vi "Host Main.vi"() -> ()   [LabVIEW 2013]
doc: "This application launches and executes the Tag Bus Data framework configuration for the specified target alias. This is a simple example of the framework API functions, but may also be a suitable starting point for a Host UI or Thick Client that is running a local version of the framework."
uses:
  <vilib>/NI/Module Execution Interface/Engine Runtime/Execution States.ctl
  <vilib>/NI/Module Execution Interface/Engine Runtime/Fault.ctl
  <vilib>/NI/Tag Bus Module Framework/runtime/error classification.ctl
  <vilib>/NI/Module Execution Interface/Engine Runtime/Engine Runtime Interface.lvclass
  <vilib>/NI/Tag Bus Data Framework/Framework Configuration Classes/target runtime/PL_Target Runtime.lvclass
  <vilib>/NI/Tag Bus Module Framework/runtime/TBM module execution interface.lvclass
panel:
  out "engine status":T4(array[cluster])
  in  "file name":string="SimulatedSystem.pcfg"
  in  "stop":bool
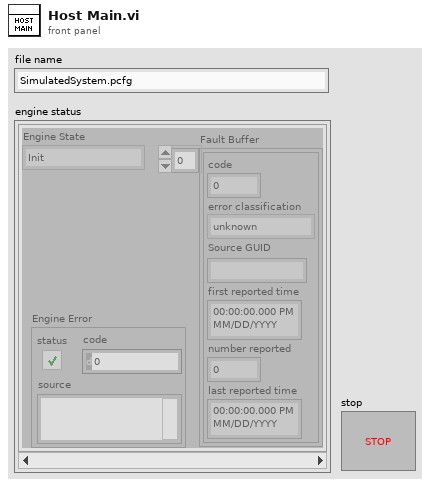
[diagram p1: front panel]
types:
  T1 = typedef "Engine Runtime Interface.lvclass/Execution States.ctl" = enum16{"Init", "Pre-Operational", "Safe-Operational", "Operational", "Stopped"}
  T2 = typedef "Engine Runtime Interface.lvclass/Fault.ctl" = cluster{"code":i32, "error classification":T3, "Source GUID":string, "first reported time":timestamp, "number reported":u32, "last reported time":timestamp}
  T3 = typedef "TBM module execution interface.lvclass/error classification.ctl" = enum16{"unknown", "none", "trivial", "recoverable", "critical"}
  T4 = cluster{"Engine State":T1, "Fault Buffer":T2[], "Engine Error":errorcluster}[]
  T5 = cluster{"Engine State":T1, "faults":T2[], "Engine Error":errorcluster}
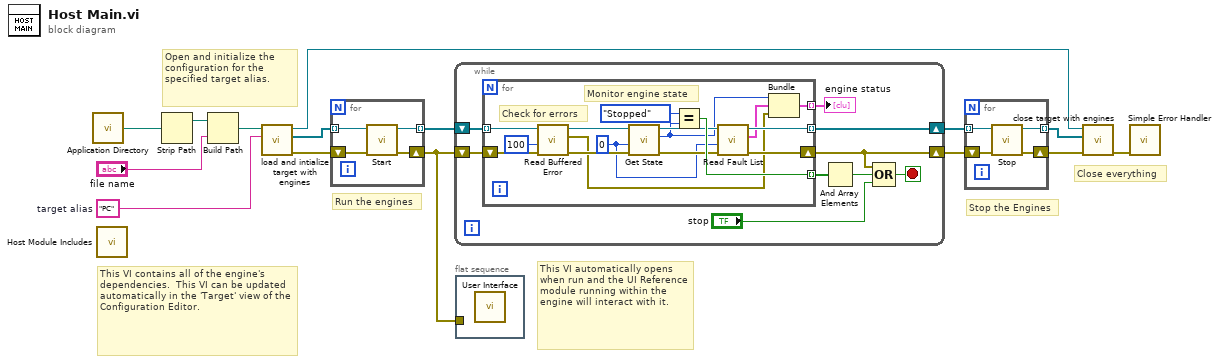
[diagram p0: block diagram]
diagram:
  w5 = "PC"  # target alias
  # "Open and initialize the configuration for the specified target alias."
  # "Close everything"
  # "Stop the Engines"
  # "This VI contains all of the engine's dependencies.  This VI can be updated automatically in the 'Target' view of the Configuration Editor."
  # "This VI automatically opens when run and the UI Reference module running within the engine will interact with it."
  # "Run the engines"
  n1 = call <vilib>:"Application Directory.vi"() -> ("Application Directory"=w11:path)
  n2 = call "Host Module Includes.vi"() -> ()  [unwired: 12 in]
  n3 = Strip Path(path=w11) -> (stripped path=w10:path)  [unwired: 1 out]
  n4 = Build Path(base path=w10, name or relative path="file name") -> (appended path=w8:path)
  n5 = call <vilib>:"load and intialize target with engines.vi"("target alias"=w5, "file path"=w8) -> ("error out"=w7:errorcluster, "engine runtime interfaces"=w6:refnum<class "Engine Runtime Interface.lvclass">[], "target runtime"=w3:refnum<class "PL_Target Runtime.lvclass">)  [unwired: 7 in]
  n6 = for {
    tunnel: [w19] -> w15 mode=indexing
    tunnel: w6 -> [w16] mode=indexing
    shift-right: [w18] -> w9
    shift-left: w7 -> [w17]
    n7 = call-dynamic "Start.vi"("error in"=w17, "Engine Runtime Interface in"=w16) -> ("error out"=w18:errorcluster, "Engine Runtime Interface out"=w19:refnum<class "Engine Runtime Interface.lvclass">)  [unwired: 8 in]
  }
  n8 = while {
    shift-right: [w26] -> w14
    shift-left: w15 -> [w28]
    shift-right: [w23] -> w13
    shift-left: w9 -> [w27]
    stop <- w24 stop-if-true
    n9 = for {
      tunnel: w28 -> [w44] mode=indexing
      tunnel: [w35] -> w26 mode=indexing
      tunnel: [w39] -> w21 mode=indexing
      shift-right: [w34] -> w23
      shift-left: w27 -> [w43]
      tunnel: [w29] -> w22 mode=indexing
      w33 = 0 ("timeout (-1)")
      # "Monitor engine state"
      # "Check for errors"
      n10 = call-dynamic "Read Buffered Error.vi"("error in"=w43, "timeout in ms (0)"=100, "Engine Runtime Interface in"=w44) -> ("error out"=w41:errorcluster, "Engine Error"=w30:errorcluster, "Engine Runtime Interface out"=w42:refnum<class "Engine Runtime Interface.lvclass">)  [unwired: 6 in]
      n11 = call-dynamic "Get State.vi"("error in"=w41, "timeout (-1)"=w33, "Engine Runtime Interface in"=w42) -> ("error out"=w37:errorcluster, "Engine State"=w32:T1, "Engine Runtime Interface out"=w36:refnum<class "Engine Runtime Interface.lvclass">)  [unwired: 6 in]
      n12 = Equal?(x=Execution_States."Stopped" ("Engine State"), y=w32) -> (x = y?=w39:bool)
      n13 = call-dynamic "Read Fault List.vi"("error in"=w37, "timeout (-1)"=w33, "Engine Runtime Interface in"=w36) -> ("error out"=w34:errorcluster, "faults"=w31:T2[], "Engine Runtime Interface out"=w35:refnum<class "Engine Runtime Interface.lvclass">)  [unwired: 6 in]
      n14 = Bundle("Engine State"=w32, "faults"=w31, "Engine Error"=w30) -> (w29:T5)  [unwired: 1 in]
    }
    "engine status" <- w22
    n15 = And Array Elements(Boolean array=w21) -> (logical AND=w20:bool)
    n16 = Compound Arithmetic op=OR(w23, w20, "stop") -> (w24:bool)
  }
  n17 = flat-sequence {
    tunnel: w9 -> [_]
    frame #0 {
      n18 = call "User Interface.vi"() -> ()  [unwired: 12 in]
    }
  }
  n19 = for {
    tunnel: w14 -> [w48] mode=indexing
    shift-right: [w45] -> w2
    shift-left: w13 -> [w47]
    tunnel: [w46] -> w4 mode=indexing
    n20 = call-dynamic "Stop.vi"("error in"=w47, "Engine Runtime Interface in"=w48) -> ("error out"=w45:errorcluster, "Engine Runtime Interface out"=w46:refnum<class "Engine Runtime Interface.lvclass">)  [unwired: 8 in]
  }
  n21 = call <vilib>:"close target with engines.vi"("error in"=w2, "Engine Runtime Interfaces"=w4, "Target Runtime"=w3) -> ("error out"=w1:errorcluster)  [unwired: 8 in]
  n22 = call <vilib>:"Simple Error Handler.vi"("error in (no error)"=w1) -> ()  [unwired: 4 in, 5 out]
